vi "_CSMOFGV.vi"(6 "Operation":T7=enum."Get By Name", 7 "Allowed Messages (Empty For All)":string[](array[string]), 8 "Error In":errorcluster caption="error in (no error)", 9 "Mode":T1, 10 "Reference":string, 11 "Name (\"\" to Use UUID) In":string) -> (0 "error out":errorcluster, 1 "Boolean":bool, 3 "Array":T2[](array[typedef]))   [LabVIEW 2017, in "Communicable State Machine.lvlib"]
uses:
  Communicable State Machine.lvlib
  _CSMOFGVOPER.ctl
  _CSMObj.ctl
  _CSMObj-Info.ctl
  Typedef/_CSM_MODE.ctl
  _CSMObj-Refs.ctl
  _CSMObj-Data.ctl
  Priority Queue/Priority Queue.ctl
  Typedef/_Cross CSM State Data.ctl
  Typedef/_CSM_MSG_TYPE.ctl
  Typedef/_Cross CSM State Response.ctl
  Typedef/_CSM_Response Source Message.ctl
  Priority Queue/def-Data(LowPRI-Q).ctl
  _CSMObj-ModeData.ctl
  Typedef/_CSM Status Change Event Data.ctl
  Typedef/_CSM_List Module Scope.ctl
  Def-CSMOMgr.ctl
  ChangeFlag/ChangeFlag-Write.vi
  Utility/Random Change Flag.vi
  ChangeFlag/ChangeFlagDB.vi
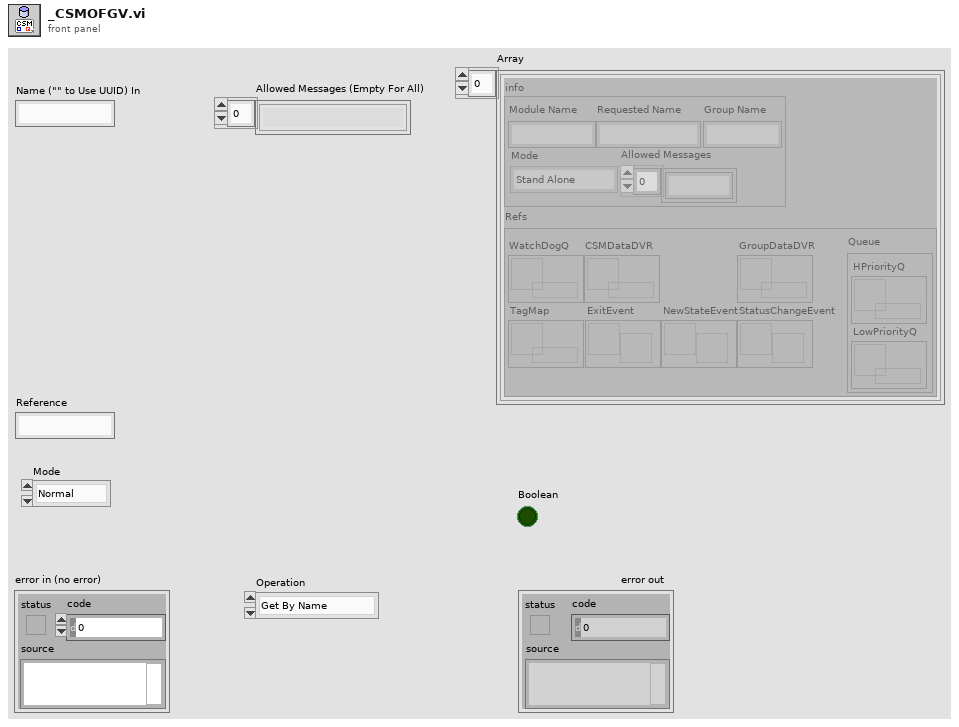
[diagram p1: front panel]
types:
  T1 = typedef "Communicable State Machine.lvlib/_CSM_List Module Scope.ctl" = enum16{"Normal", "System Only", "All"}
  T2 = typedef "Communicable State Machine.lvlib/_CSMObj.ctl" = cluster{"info":T3, "Refs":T5}
  T3 = typedef "Communicable State Machine.lvlib/_CSMObj-Info.ctl" = cluster{"Module Name":string, "Requested Name":string, "Group Name":string, "Mode":T4, "Allowed Messages":string[]}
  T4 = typedef "Communicable State Machine.lvlib/_CSM_MODE.ctl" = enum16{"Not Exist", "Stand Alone", "CSM", "Worker", "Worker Agent", "Chain Node", "Chain"}
  T5 = typedef "Communicable State Machine.lvlib/_CSMObj-Refs.ctl" = cluster{"WatchDogQ":refnum<queue>, "CSMDataDVR":refnum<data-value>, "Queue":T6, "GroupDataDVR":refnum<data-value>, "TagMap":refnum<data-value>, "ExitEvent":refnum<user-event>, "NewStateEvent":refnum<user-event>, "StatusChangeEvent":refnum<user-event>}
  T6 = typedef "Communicable State Machine.lvlib/Priority Queue.ctl" = cluster{"HPriorityQ":refnum<queue>, "LowPriorityQ":refnum<queue>}
  T7 = typedef "Communicable State Machine.lvlib/_CSMOFGVOPER.ctl" = enum16{"Create If not Exist", "Get By Name", "List", "Check If Name Exists", "Release", "Module Status", "Create Status Event Handler", "Destroy Status Event Handler", "Clear Invalid Objs"}
  T8 = typedef "Communicable State Machine.lvlib/Def-CSMOMgr.ctl" = variant
  T9 = typedef "Communicable State Machine.lvlib/_CSMObj-ModeData.ctl" = cluster{"CSMDataDVR":refnum<data-value>[], "Messages of Chain Nodes":cluster{"Module Name":string, "Allowed Messages":string[]}[], "Chain Message Mapping Map":variant}
  T10 = cluster{"Module Name":string, "Allowed Messages":string[]}[]
  T11 = cluster{"Module Name":string, "Allowed Messages":string[]}
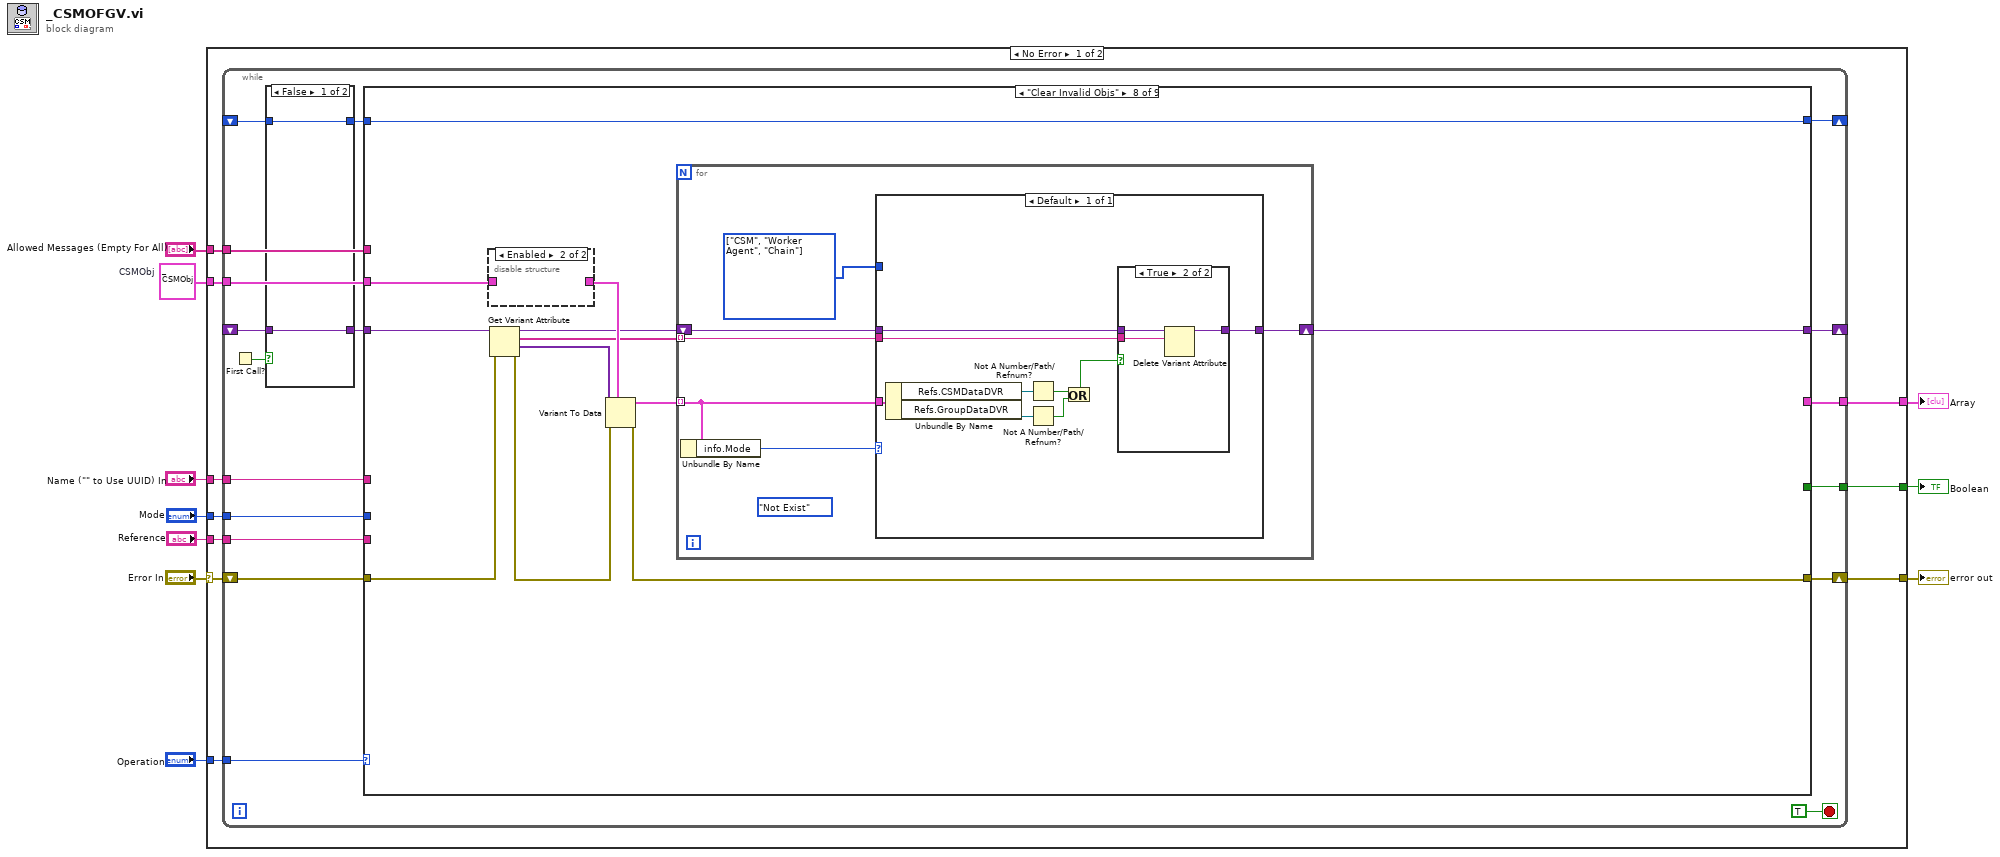
[diagram p0: block diagram]
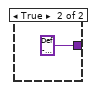
[diagram p2: hidden frame]
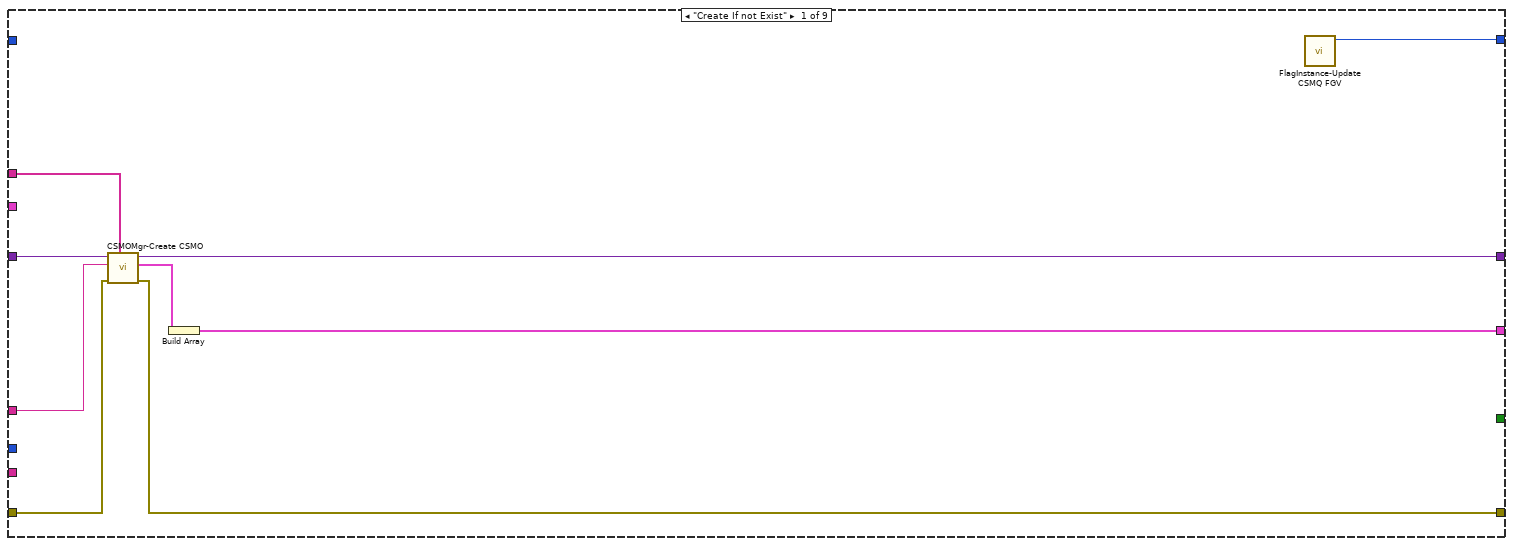
[diagram p3: hidden frame]
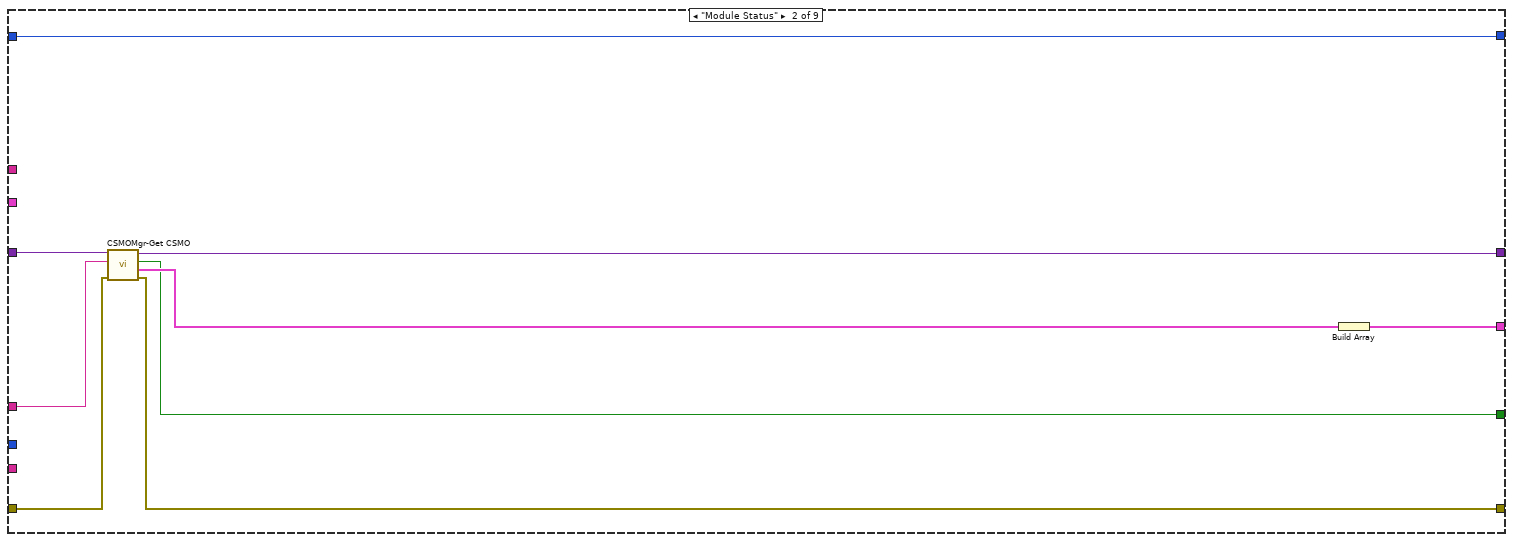
[diagram p4: hidden frame]
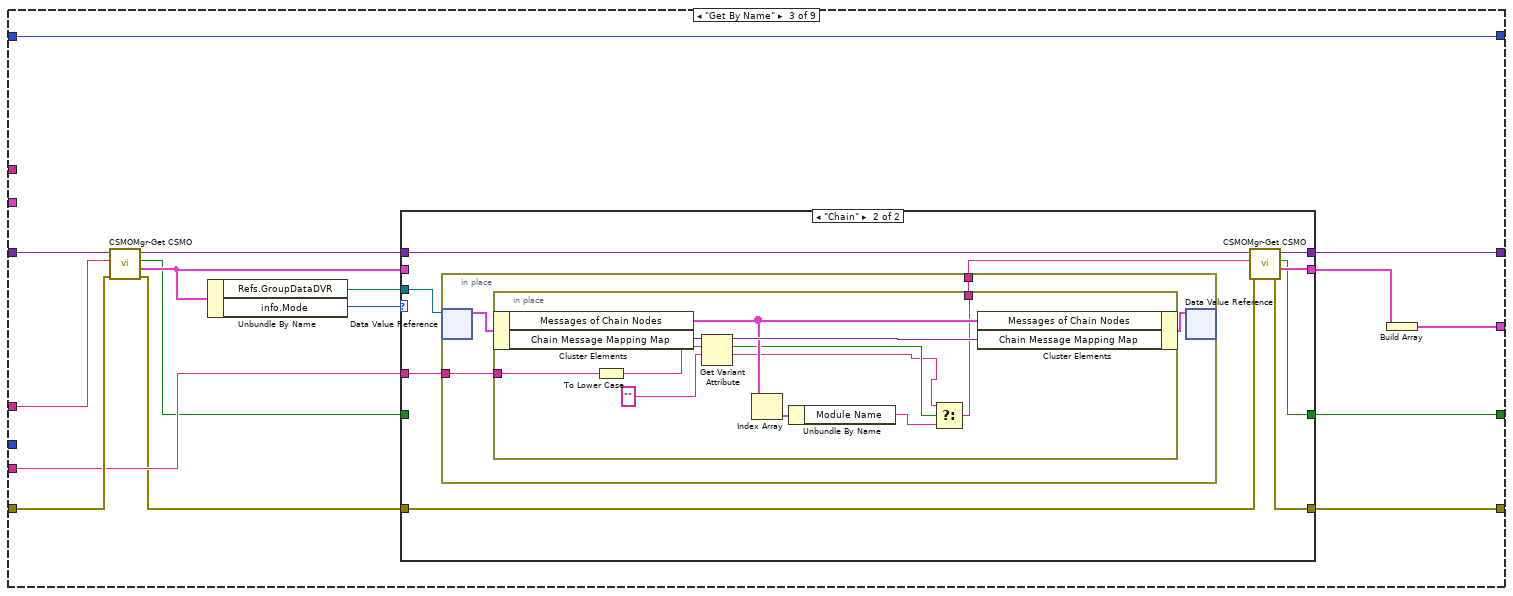
[diagram p5: hidden frame]
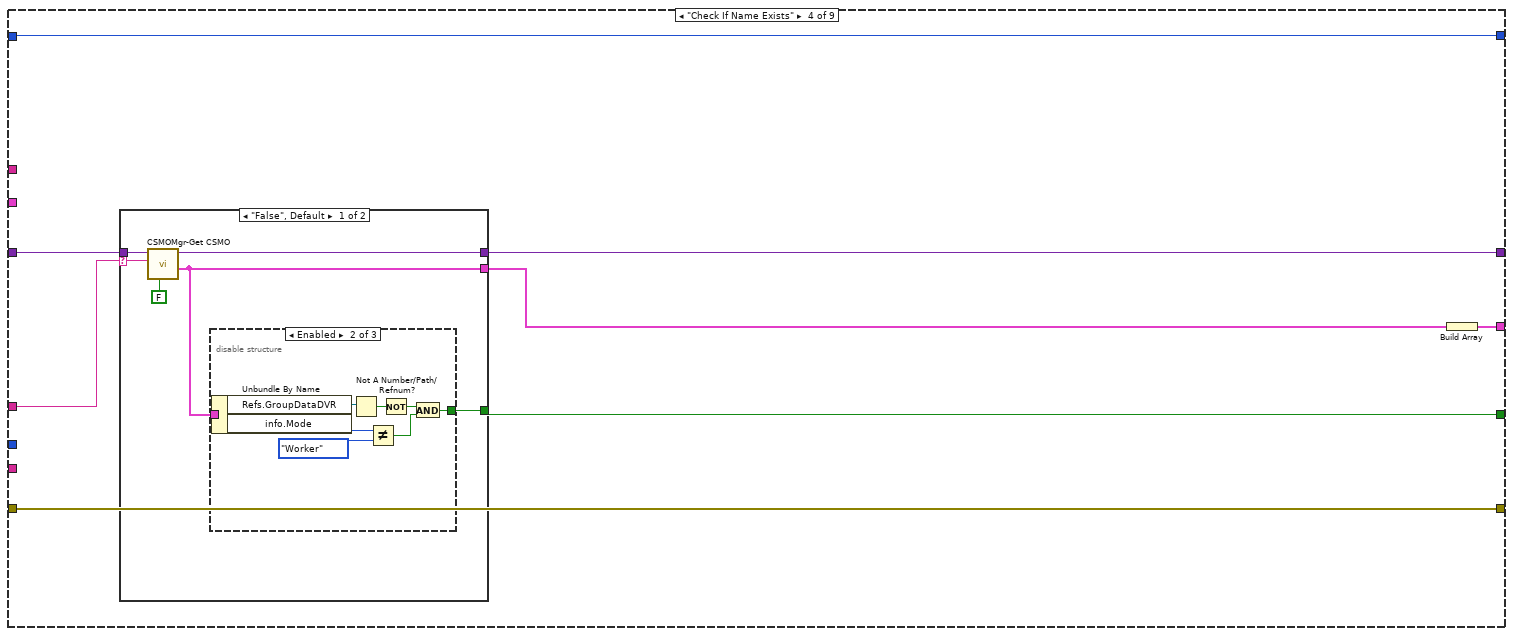
[diagram p7: hidden frame]
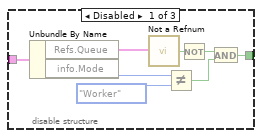
[diagram p8: hidden frame]
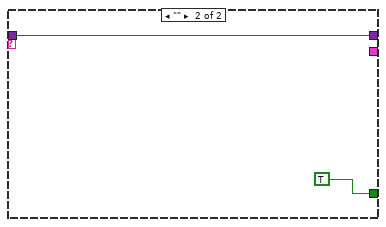
[diagram p10: hidden frame]
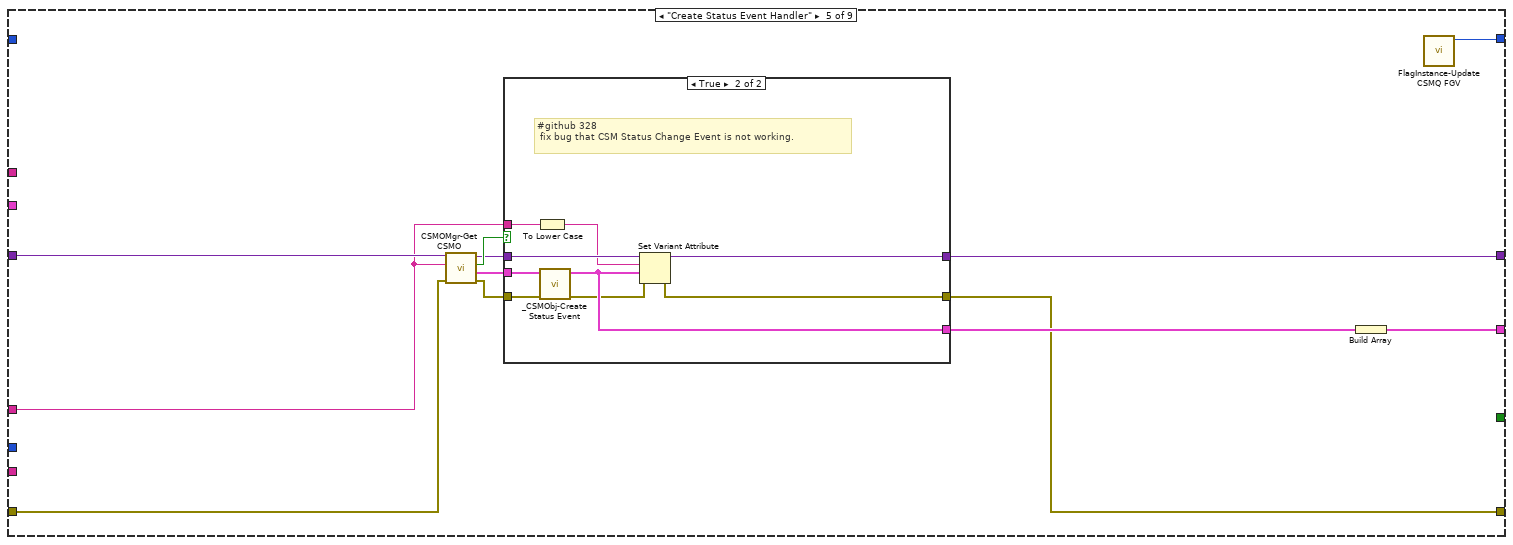
[diagram p11: hidden frame]
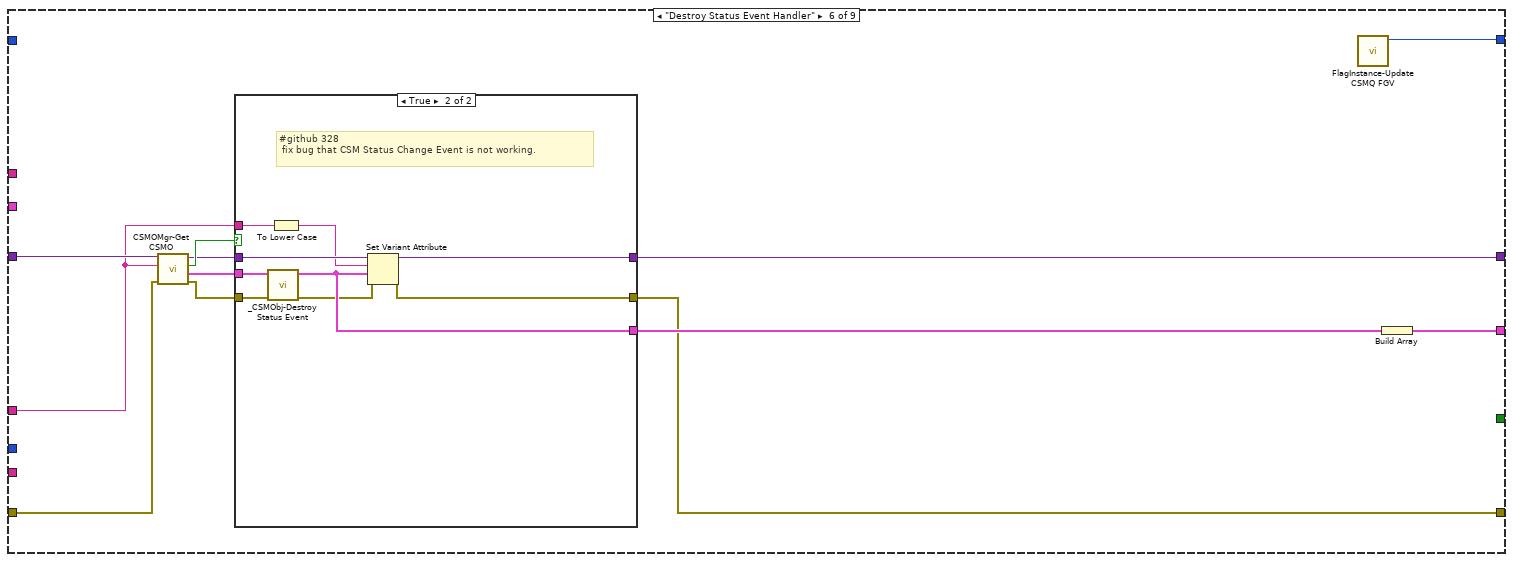
[diagram p13: hidden frame]
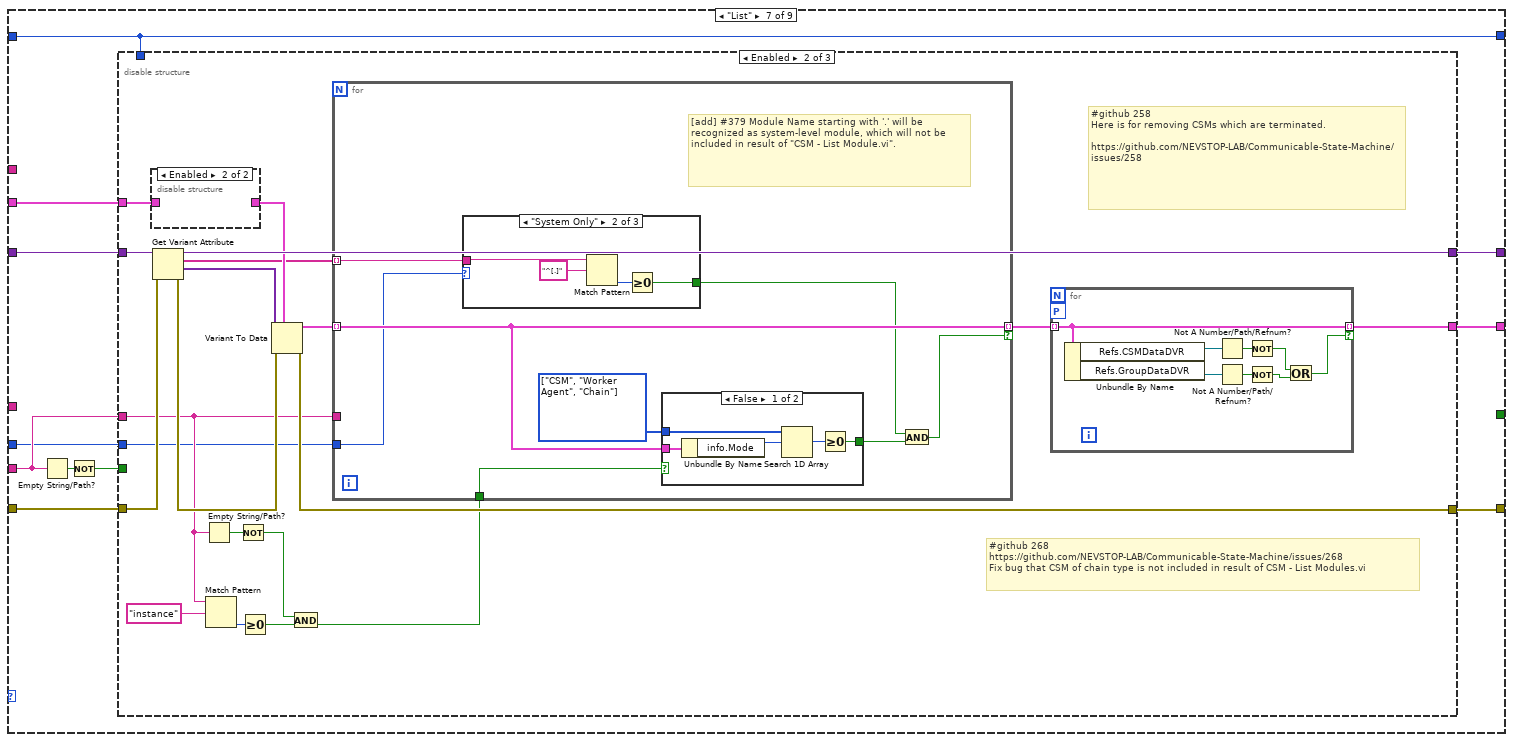
[diagram p15: hidden frame]
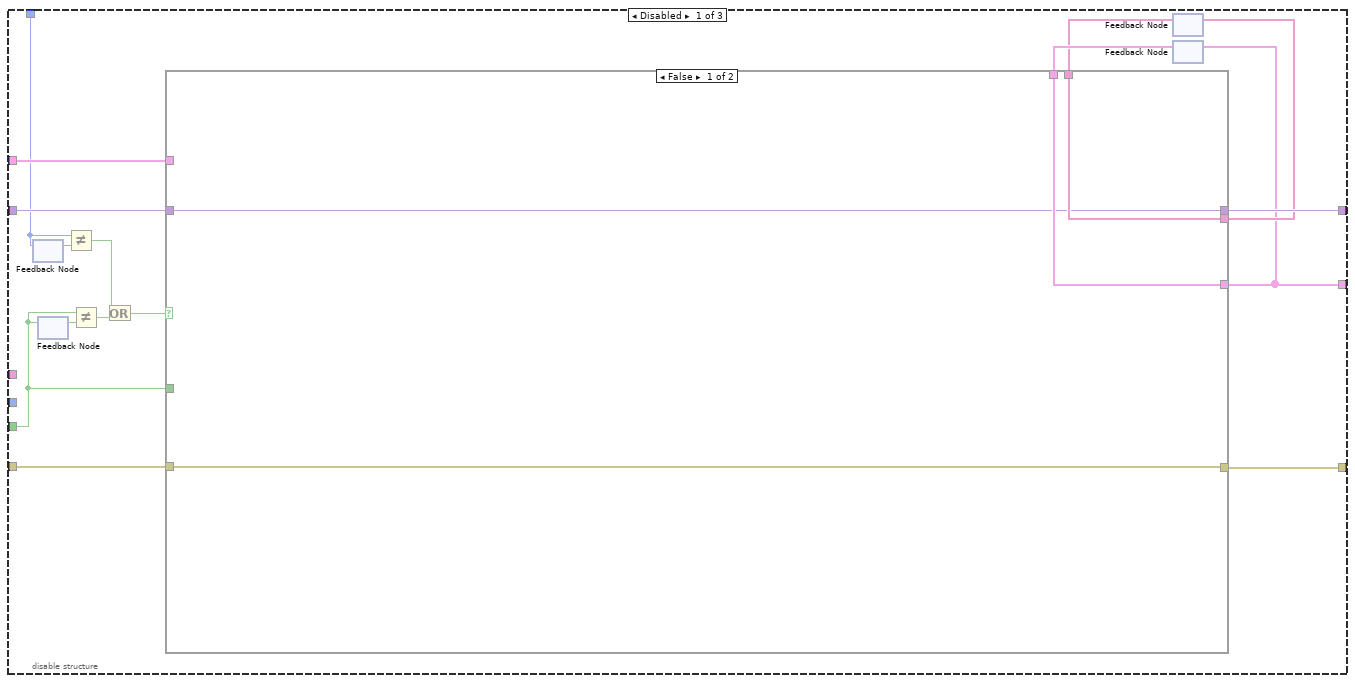
[diagram p16: hidden frame]
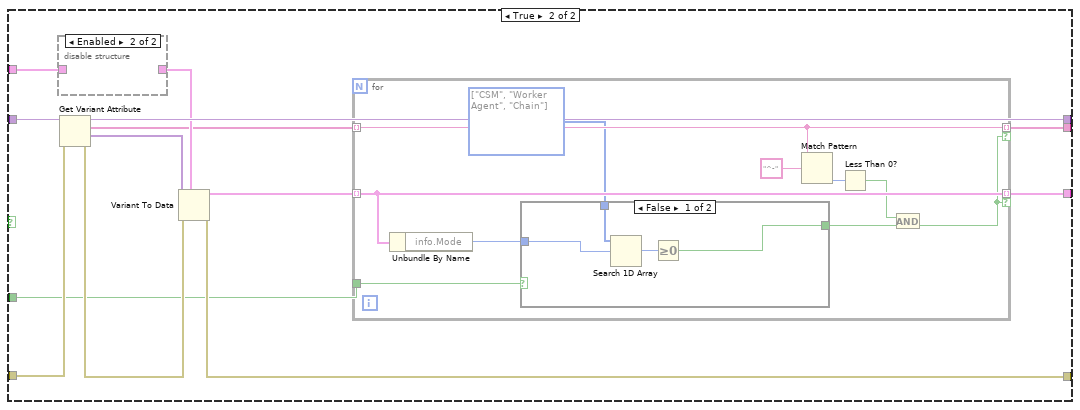
[diagram p17: hidden frame]
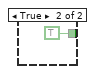
[diagram p18: hidden frame]
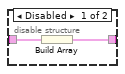
[diagram p19: hidden frame]
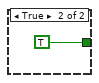
[diagram p20: hidden frame]
diagram:
  w6 = T2 {"info"={"Module Name"="", "Requested Name"="", "Group Name"="", "Mode"=enum."Stand Alone", "Allowed Messages"=[]}, "Refs"={"WatchDogQ"=refnum, "CSMDataDVR"=refnum, "Queue"={"HPriorityQ"=refnum, "LowPriorityQ"=refnum}, "GroupDataDVR"=refnum, "TagMap"=refnum, "ExitEvent"=refnum, "NewStateEvent"=refnum, "StatusChangeEvent"=refnum}}  # CSMObj
  n1 = case shown="No Error" "Error In" {
    selector: "Error In" -> [w18 w337]
    tunnel: "Operation" -> [w20 _]
    tunnel: "Name (\"\" to Use UUID) In" -> [w19 _]
    tunnel: [w17 w337] -> w7
    tunnel: w6 -> [w16 _]
    tunnel: [w15 _] -> w5
    tunnel: [w14 _] -> w4
    tunnel: "Allowed Messages (Empty For All)" -> [w13 _]
    tunnel: "Reference" -> [w12 _]
    tunnel: "Mode" -> [w11 _]
    frame No Error {
      n2 = while {
        tunnel: w20 -> [w37]
        tunnel: w19 -> [w36]
        tunnel: [w35] -> w15
        shift-right: [w31] -> _
        shift-left: _ -> [w33]
        shift-right: [w29] -> w17
        shift-left: w18 -> [w30]
        tunnel: w16 -> [w28]
        tunnel: [w27] -> w14
        shift-right: [w26] -> _
        shift-left: _ -> [w24]
        tunnel: w13 -> [w23]
        tunnel: w12 -> [w22]
        tunnel: w11 -> [w21]
        stop <- TRUE stop-if-true
        n3 = First Call?() -> (First Call?: T/F=w34:bool)
        n4 = case shown="False" w34 {
          tunnel: [w40 T8 variant] -> w32
          tunnel: w33 -> [w40 _]
          tunnel: [w39 _] -> w25
          tunnel: w24 -> [w39 _]
          frame False {
          }
          frame True {
          }
        }
        n5 = case shown="\"Clear Invalid Objs\"" w37 {
          tunnel: w36 -> [w43 w51 w71 w104 w146 w170 _ _ w334]
          tunnel: [w46 w56 w74 w108 w140 w164 w188 _ _] -> w35
          tunnel: w32 -> [w44 w59 w75 w105 w147 w171 w194 w309 w336]
          tunnel: [w50 w58 w67 w111 w142 w166 w193 w298 w333] -> w31
          tunnel: w30 -> [w47 w54 w72 w109 w139 w163 w191 w307 w335]
          tunnel: [w49 w53 w60 w109 w137 w161 w190 w306 w332] -> w29
          tunnel: w28 -> [_ _ _ _ _ _ w192 w308 _]
          tunnel: [_ w52 w61 w107 _ _ _ _ _] -> w27
          tunnel: w25 -> [_ w55 w73 w106 _ _ w189 w305 _]
          tunnel: [w42 w55 w73 w106 w136 w160 w189 w305 w331] -> w26
          tunnel: w23 -> [w45 _ _ _ _ _ _ _ _]
          tunnel: w22 -> [_ _ w65 _ _ _ w185 _ _]
          tunnel: w21 -> [_ _ _ _ _ _ w184 _ _]
          frame "Create If not Exist" {
            n6 = call "CSMOMgr-Create CSMO.vi"("Allowed Messages (Empty For All)"=w45, "error in (no error)"=w47, "Name (\"\" to Use UUID) In"=w43, "CSMOMgr"=w44) -> ("error out"=w49:errorcluster, "CSMO"=w48:T2, "CSMOMgr Out"=w50:T8)  [unwired: 5 in]
            n7 = Build Array(w48) -> (w46:T2[])
            n8 = call "FlagInstance-Update CSMQ FGV.vi"() -> ("New Random Change Flag"=w42:u64)  [unwired: 10 in, 1 out]
          }
          frame "Module Status" {
            n9 = call "CSMOMgr-Get CSMO.vi"("Error In"=w54, "Queue Name"=w51, "CSMOMgr"=w59) -> ("error out"=w53:errorcluster, "Values"=w57:T2, "Found"=w52:bool, "CSMOMgr Out"=w58:T8)  [unwired: 5 in]
            n10 = Build Array(w57) -> (w56:T2[])
          }
          frame "Get By Name" {
            n11 = call "CSMOMgr-Get CSMO.vi"("Error In"=w72, "Queue Name"=w71, "CSMOMgr"=w75) -> ("error out"=w63:errorcluster, "Values"=w69:T2, "Found"=w62:bool, "CSMOMgr Out"=w66:T8)  [unwired: 5 in]
            n12 = Unbundle By Name(w69) -> ("Refs.GroupDataDVR"=w64:refnum<data-value>, "info.Mode"=w70:T4)
            n13 = case shown="\"Chain\"" w70 {
              tunnel: w69 -> [w79 _]
              tunnel: [w79 w86] -> w68
              tunnel: [w78 w81] -> w67
              tunnel: w66 -> [w78 w82]
              tunnel: w65 -> [_ w87]
              tunnel: w64 -> [_ w88]
              tunnel: w63 -> [w76 w84]
              tunnel: w62 -> [w77 _]
              tunnel: [w77 w85] -> w61
              tunnel: [w76 w83] -> w60
              frame "Not Exist", Default {
              }
              frame "Chain" {
                n14 = in-place {
                  in-place-border: w87 -> [w90]
                  in-place-border: [w89] -> w80
                  n15 = in-place-dvr #1(w88) -> (w92:T9)  [unwired: 1 out]
                  n16 = in-place {
                    in-place-border: w90 -> [w101]
                    in-place-border: [w95] -> w89
                    n17 = in-place-cluster #2(w92) -> ("Messages of Chain Nodes"=w98:T10, "Chain Message Mapping Map"=w103:variant)
                    n18 = To Lower Case(string=w101) -> (all lower case string=w99:string)
                    n19 = Get Variant Attribute(Variant=w103, name=w99, default value (empty Variant)="") -> (duplicate Variant=w102:variant, found=w96:bool, value=w94:string)  [unwired: 1 in, 1 out]
                    n20 = Index Array(array=w98) -> (element=w97:T11)  [unwired: 1 in]
                    n21 = Unbundle By Name(w97) -> ("Module Name"=w93:string)
                    n22 = Select(t=w94, s=w96, f=w93) -> (s? t:f=w95:string)
                    n23 = in-place-cluster #2("Messages of Chain Nodes"=w98, "Chain Message Mapping Map"=w102) -> (w91:T9)
                  }
                  n24 = in-place-dvr #1(w91) -> ()  [unwired: 2 out]
                }
                n25 = call "CSMOMgr-Get CSMO.vi"("Error In"=w84, "Queue Name"=w80, "CSMOMgr"=w82) -> ("error out"=w83:errorcluster, "Values"=w86:T2, "Found"=w85:bool, "CSMOMgr Out"=w81:T8)  [unwired: 5 in]
              }
            }
            n26 = Build Array(w68) -> (w74:T2[])
          }
          frame "Check If Name Exists" {
            n27 = case shown="\"False\", Default" w104 {
              selector: w104 -> [w114 _]
              tunnel: w105 -> [w116 w135]
              tunnel: [w115 w135] -> w111
              tunnel: [w113 _] -> w110
              tunnel: [w117 TRUE] -> w107
              frame "False", Default {
                n28 = call "CSMOMgr-Get CSMO.vi"("GenError? (T)"=FALSE ("GenError?(T)"), "Queue Name"=w114, "CSMOMgr"=w116) -> ("Values"=w113:T2, "CSMOMgr Out"=w115:T8)  [unwired: 5 in, 2 out]
                n29 = disable-structure shown="Enabled" {
                  disable-tunnel: [w122 w130 _] -> w117
                  disable-tunnel: w113 -> [w118 w126 _]
                  frame Disabled {
                    n30 = Unbundle By Name(w118) -> ("Refs.Queue"=w125:T6, "info.Mode"=w121:T4)
                    n31 = call "Not a Refnum.vi"("Priority Queue.lvclass"=w125) -> ("NaN/Path/Refnum?"=w124:bool)  [unwired: 4 in]
                    n32 = Not Equal?(x=w121, y=_CSM_MODE."Worker") -> (x != y?=w119:bool)
                    n33 = Not(x=w124) -> (.not. x?=w123:bool)
                    n34 = And(x=w123, y=w119) -> (x .and. y?=w122:bool)
                  }
                  frame Enabled {
                    n35 = Unbundle By Name(w126) -> ("Refs.GroupDataDVR"=w133:refnum<data-value>, "info.Mode"=w129:T4)
                    n36 = Not A Number/Path/Refnum?(number/path/refnum=w133) -> (NaN/Path/Refnum?=w132:bool)
                    n37 = Not Equal?(x=w129, y=_CSM_MODE."Worker") -> (x != y?=w127:bool)
                    n38 = Not(x=w132) -> (.not. x?=w131:bool)
                    n39 = And(x=w131, y=w127) -> (x .and. y?=w130:bool)
                  }
                  frame Disabled {
                  }
                }
              }
              frame "" {
              }
            }
            n40 = Build Array(w110) -> (w108:T2[])
          }
          frame "Create Status Event Handler" {
            n41 = call "CSMOMgr-Get CSMO.vi"("Error In"=w139, "Queue Name"=w146, "CSMOMgr"=w147) -> ("error out"=w138:errorcluster, "Values"=w145:T2, "Found"=w144:bool, "CSMOMgr Out"=w143:T8)  [unwired: 5 in]
            n42 = case shown="True" w144 {
              tunnel: w145 -> [w149 w156]
              tunnel: w143 -> [w150 w159]
              tunnel: [w150 w158] -> w142
              tunnel: w146 -> [_ w157]
              tunnel: [w149 w155] -> w141
              tunnel: w138 -> [w148 w154]
              tunnel: [w148 w152] -> w137
              frame False {
              }
              frame True {
                # "#github 328\n fix bug that CSM Status Change Event is not working."
                n43 = To Lower Case(string=w157) -> (all lower case string=w151:string)
                n44 = call "_CSMObj-Create Status Event.vi"("Error In"=w154, "Values In"=w156) -> ("error out"=w153:errorcluster, "Values Out"=w155:T2)  [unwired: 8 in]
                n45 = Set Variant Attribute(Variant=w159, name=w151, value=w155, error in=w153) -> (Variant out=w158:T8, error out=w152:errorcluster)  [unwired: 1 out]
              }
            }
            n46 = Build Array(w141) -> (w140:T2[])
            n47 = call "FlagInstance-Update CSMQ FGV.vi"() -> ("New Random Change Flag"=w136:u64)  [unwired: 10 in, 1 out]
          }
          frame "Destroy Status Event Handler" {
            n48 = call "CSMOMgr-Get CSMO.vi"("Error In"=w163, "Queue Name"=w170, "CSMOMgr"=w171) -> ("error out"=w162:errorcluster, "Values"=w169:T2, "Found"=w168:bool, "CSMOMgr Out"=w167:T8)  [unwired: 5 in]
            n49 = case shown="True" w168 {
              tunnel: w169 -> [w173 w180]
              tunnel: w167 -> [w174 w183]
              tunnel: [w174 w182] -> w166
              tunnel: w170 -> [_ w181]
              tunnel: [w173 w179] -> w165
              tunnel: w162 -> [w172 w178]
              tunnel: [w172 w176] -> w161
              frame False {
              }
              frame True {
                # "#github 328\n fix bug that CSM Status Change Event is not working."
                n50 = call "_CSMObj-Destroy Status Event.vi"("Error In"=w178, "Values In"=w180) -> ("error out"=w177:errorcluster, "Values Out"=w179:T2)  [unwired: 8 in]
                n51 = To Lower Case(string=w181) -> (all lower case string=w175:string)
                n52 = Set Variant Attribute(Variant=w183, name=w175, value=w179, error in=w177) -> (Variant out=w182:T8, error out=w176:errorcluster)  [unwired: 1 out]
              }
            }
            n53 = call "FlagInstance-Update CSMQ FGV.vi"() -> ("New Random Change Flag"=w160:u64)  [unwired: 10 in, 1 out]
            n54 = Build Array(w165) -> (w164:T2[])
          }
          frame "List" {
            n55 = Empty String/Path?(string/path=w185) -> (empty?=w187:bool)
            n56 = Not(x=w187) -> (.not. x?=w186:bool)
            n57 = disable-structure shown="Enabled" {
              disable-tunnel: w194 -> [w210 w264 _]
              disable-tunnel: [w209 w263 _] -> w193
              disable-tunnel: w192 -> [w208 w262 _]
              disable-tunnel: w191 -> [w207 w261 _]
              disable-tunnel: [w206 w260 _] -> w190
              disable-tunnel: w189 -> [w204 _ _]
              disable-tunnel: [w198 w253 _] -> w188
              disable-tunnel: w186 -> [w195 _ _]
              disable-tunnel: w185 -> [_ w247 _]
              disable-tunnel: w184 -> [_ w245 _]
              frame Disabled {
                n58 = feedback #3() -> (w205:u64)  [unwired: 1 in]
                n59 = feedback-in #3(w204) -> ()
                n60 = feedback #4() -> (w203:bool)  [unwired: 1 in]
                n61 = feedback-in #4(w195) -> ()
                n62 = Not Equal?(x=w204, y=w205) -> (x != y?=w201:bool)
                n63 = Not Equal?(x=w195, y=w203) -> (x != y?=w202:bool)
                n64 = Or(x=w201, y=w202) -> (x .or. y?=w200:bool)
                n65 = feedback #5() -> (w196:string[])  [unwired: 1 in]
                n66 = feedback #6() -> (w197:T2[])  [unwired: 1 in]
                n67 = case shown="False" w200 {
                  tunnel: w210 -> [w212 w227]
                  tunnel: [w212 w226] -> w209
                  tunnel: w208 -> [_ w224]
                  tunnel: [w213 w220] -> w199
                  tunnel: [w214 w219] -> w198
                  tunnel: w207 -> [w211 w217]
                  tunnel: [w211 w216] -> w206
                  tunnel: w195 -> [_ w215]
                  tunnel: w197 -> [w214 _]
                  tunnel: w196 -> [w213 _]
                  frame False {
                  }
                  frame True {
                    n68 = disable-structure shown="Enabled" {
                      disable-tunnel: w224 -> [w244 _]
                      disable-tunnel: [w243 _] -> w223
                      frame Disabled {
                        n69 = Build Array(w244) -> (w243:T2[])
                      }
                      frame Enabled {
                      }
                    }
                    n70 = Get Variant Attribute(Variant=w227, error in=w217) -> (duplicate Variant=w226:variant, names=w221:string[], values=w225:variant[], error out=w218:errorcluster)  [unwired: 2 in]
                    n71 = Variant To Data(error in=w218, type=w223, Variant=w225) -> (data=w222:T2[], error out=w216:errorcluster)
                    n72 = for {
                      tunnel: w222 -> [w237] mode=indexing
                      tunnel: w221 -> [w232] mode=indexing
                      tunnel: [w232] -> w220 mode=indexing if=w233
                      tunnel: [w237] -> w219 mode=indexing if=w233
                      tunnel: w215 -> [w234]
                      w228 = T4[] [enum."CSM", enum."Worker Agent", enum."Chain"] items=["Not Exist", "Stand Alone", "CSM", "Worker", "Worker Agent", "Chain Node", "Chain"]
                      n73 = Unbundle By Name(w237) -> ("info.Mode"=w236:T4)
                      n74 = case shown="False" w234 {
                        tunnel: [w238 TRUE] -> w235
                        tunnel: w236 -> [w241 _]
                        tunnel: w228 -> [w240 _]
                        frame False {
                          n75 = Search 1D Array(1D array=w240, element=w241) -> (index of element=w239:i32)  [unwired: 1 in]
                          n76 = Greater Or Equal To 0?(x=w239) -> (x >= 0?=w238:bool)
                        }
                        frame True {
                        }
                      }
                      n77 = Match Pattern(string=w232, regular expression="^-") -> (offset past match=w230:i32)  [unwired: 1 in, 3 out]
                      n78 = Less Than 0?(x=w230) -> (x < 0?=w229:bool)
                      n79 = And(x=w229, y=w235) -> (x .and. y?=w233:bool)
                    }
                  }
                }
                n80 = feedback-in #5(w199) -> ()
                n81 = feedback-in #6(w198) -> ()
              }
              frame Enabled {
                # "#github 268\nhttps://github.com/NEVSTOP-LAB/Communicable-State-Machine/issues/268\nFix bug that CSM of chain type is not included in result of CSM - List Modules.vi"
                # "#github 258\nHere is for removing CSMs which are terminated.\n\nhttps://github.com/NEVSTOP-LAB/Communicable-State-Machine/issues/258"
                n82 = disable-structure shown="Enabled" {
                  disable-tunnel: w262 -> [w297 _]
                  disable-tunnel: [w296 _] -> w258
                  frame Disabled {
                    n83 = Build Array(w297) -> (w296:T2[])
                  }
                  frame Enabled {
                  }
                }
                n84 = Get Variant Attribute(Variant=w264, error in=w261) -> (duplicate Variant=w263:variant, names=w256:string[], values=w259:variant[], error out=w255:errorcluster)  [unwired: 2 in]
                n85 = Empty String/Path?(string/path=w247) -> (empty?=w248:bool)
                n86 = Match Pattern(string=w247, regular expression="instance") -> (offset past match=w251:i32)  [unwired: 1 in, 3 out]
                n87 = Not(x=w248) -> (.not. x?=w246:bool)
                n88 = Greater Or Equal To 0?(x=w251) -> (x >= 0?=w250:bool)
                n89 = Variant To Data(error in=w255, type=w258, Variant=w259) -> (data=w257:T2[], error out=w260:errorcluster)
                n90 = And(x=w246, y=w250) -> (x .and. y?=w249:bool)
                n91 = for {
                  tunnel: w257 -> [w280] mode=indexing
                  tunnel: w256 -> [w277] mode=indexing
                  tunnel: [w280] -> w254 mode=indexing if=w278
                  tunnel: w247 -> [_]
                  tunnel: w249 -> [w274]
                  tunnel: w245 -> [w273]
                  w275 = T4[] [enum."CSM", enum."Worker Agent", enum."Chain"] items=["Not Exist", "Stand Alone", "CSM", "Worker", "Worker Agent", "Chain Node", "Chain"]
                  # "[add] #379 Module Name starting with '.' will be recognized as system-level module, which will not be included in result of \"CSM - List Module.vi\"."
                  n92 = case shown="\"System Only\"" w273 {
                    tunnel: w277 -> [w290 w294 _]
                    tunnel: [w287 w291 TRUE] -> w276
                    frame "Normal" {
                      n93 = Match Pattern(string=w290, regular expression="^[.]") -> (offset past match=w288:i32)  [unwired: 1 in, 3 out]
                      n94 = Less Than 0?(x=w288) -> (x < 0?=w287:bool)
                    }
                    frame "System Only" {
                      n95 = Match Pattern(string=w294, regular expression="^[.]") -> (offset past match=w292:i32)  [unwired: 1 in, 3 out]
                      n96 = Greater Or Equal To 0?(x=w292) -> (x >= 0?=w291:bool)
                    }
                    frame "All" {
                    }
                  }
                  n97 = case shown="False" w274 {
                    tunnel: w280 -> [w285 _]
                    tunnel: [w283 TRUE] -> w279
                    tunnel: w275 -> [w282 _]
                    frame False {
                      n98 = Unbundle By Name(w285) -> ("info.Mode"=w284:T4)
                      n99 = Search 1D Array(1D array=w282, element=w284) -> (index of element=w281:i32)  [unwired: 1 in]
                      n100 = Greater Or Equal To 0?(x=w281) -> (x >= 0?=w283:bool)
                    }
                    frame True {
                    }
                  }
                  n101 = And(x=w276, y=w279) -> (x .and. y?=w278:bool)
                }
                n102 = for {
                  tunnel: w254 -> [w265] mode=indexing
                  tunnel: [w265] -> w253 mode=indexing if=w271
                  workers-P: _ -> [_]
                  n103 = Unbundle By Name(w265) -> ("Refs.CSMDataDVR"=w268:refnum<data-value>, "Refs.GroupDataDVR"=w267:refnum<data-value>)
                  n104 = Not A Number/Path/Refnum?(number/path/refnum=w268) -> (NaN/Path/Refnum?=w272:bool)
                  n105 = Not A Number/Path/Refnum?(number/path/refnum=w267) -> (NaN/Path/Refnum?=w269:bool)
                  n106 = Not(x=w272) -> (.not. x?=w270:bool)
                  n107 = Not(x=w269) -> (.not. x?=w266:bool)
                  n108 = Or(x=w270, y=w266) -> (x .or. y?=w271:bool)
                }
              }
              frame Disabled {
              }
            }
          }
          frame "Clear Invalid Objs" {
            n109 = disable-structure shown="Enabled" {
              disable-tunnel: w308 -> [w330 _]
              disable-tunnel: [w329 _] -> w303
              frame Disabled {
                n110 = Build Array(w330) -> (w329:T2[])
              }
              frame Enabled {
              }
            }
            n111 = Get Variant Attribute(Variant=w309, error in=w307) -> (duplicate Variant=w299:variant, names=w301:string[], values=w304:variant[], error out=w300:errorcluster)  [unwired: 2 in]
            n112 = Variant To Data(error in=w300, type=w303, Variant=w304) -> (data=w302:T2[], error out=w306:errorcluster)
            n113 = for {
              tunnel: w302 -> [w313] mode=indexing
              tunnel: w301 -> [w310] mode=indexing
              shift-right: [w312] -> w298
              shift-left: w299 -> [w311]
              (unwired) _CSM_MODE."Not Exist" ("Mode")
              w314 = T4[] [enum."CSM", enum."Worker Agent", enum."Chain"] items=["Not Exist", "Stand Alone", "CSM", "Worker", "Worker Agent", "Chain Node", "Chain"]
              n114 = Unbundle By Name(w313) -> ("info.Mode"=w315:T4)
              n115 = case shown="Default" w315 {
                tunnel: w314 -> [_]
                tunnel: w313 -> [w324]
                tunnel: [w320] -> w312
                tunnel: w311 -> [w321]
                tunnel: w310 -> [w319]
                frame Default {
                  n116 = Unbundle By Name(w324) -> ("Refs.CSMDataDVR"=w323:refnum<data-value>, "Refs.GroupDataDVR"=w322:refnum<data-value>)
                  n117 = Not A Number/Path/Refnum?(number/path/refnum=w323) -> (NaN/Path/Refnum?=w318:bool)
                  n118 = Not A Number/Path/Refnum?(number/path/refnum=w322) -> (NaN/Path/Refnum?=w317:bool)
                  n119 = Or(x=w318, y=w317) -> (x .or. y?=w316:bool)
                  n120 = case shown="True" w316 {
                    tunnel: w321 -> [w325 w328]
                    tunnel: [w325 w327] -> w320
                    tunnel: w319 -> [_ w326]
                    frame False {
                    }
                    frame True {
                      n121 = Delete Variant Attribute(6:w326, 7:w328) -> (3:w327:variant)  [unwired: 1 in, 2 out]
                    }
                  }
                }
              }
            }
          }
          frame "Release" {
            n122 = call "CSMOMgr-Delete CSMO.vi"("Error In"=w335, "Queue Name"=w334, "CSMOMgr"=w336) -> ("error out"=w332:errorcluster, "CSMOMgr Out"=w333:T8)  [unwired: 7 in]
            n123 = call "FlagInstance-Update CSMQ FGV.vi"() -> ("New Random Change Flag"=w331:u64)  [unwired: 10 in, 1 out]
          }
        }
      }
    }
    frame Error {
    }
  }
  "error out" <- w7
  "Array" <- w5
  "Boolean" <- w4
